vi "Carica lista canali.vi"(9 "BANCO":i32, 10 "LINEA":i32, 11 "Array":refnum<vi>[](array[refnum])) -> (0 "error out":errorcluster)   [LabVIEW 2019]
uses:
  <vilib>/Utility/file.llb/Read Delimited Spreadsheet (string).vi
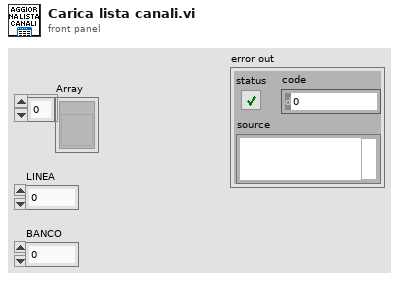
[diagram p1: front panel]
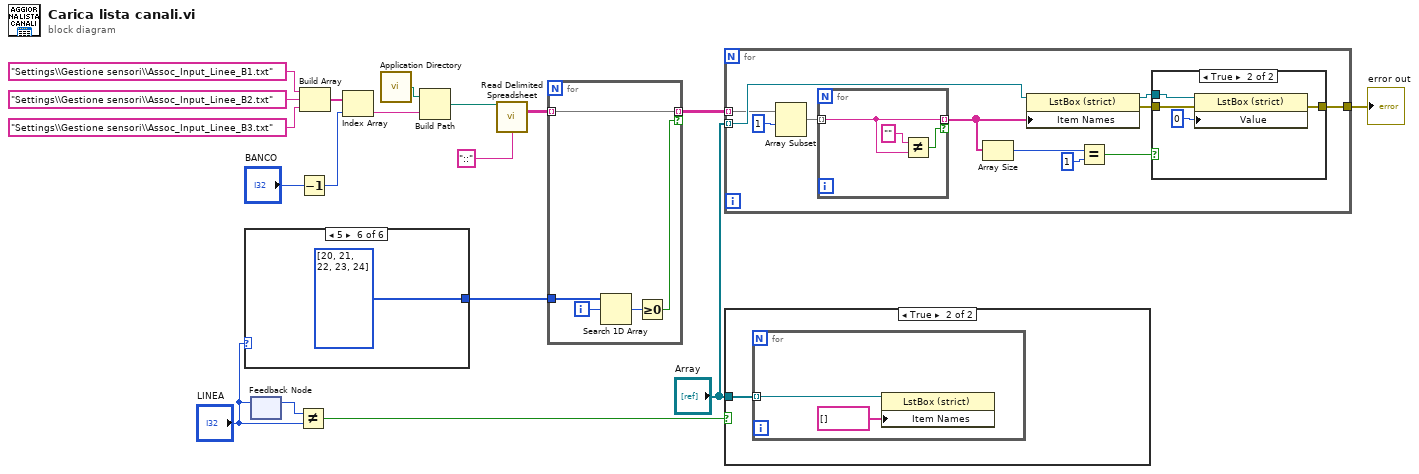
[diagram p0: block diagram]
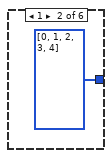
[diagram p4: hidden frame]
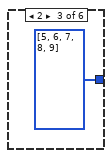
[diagram p5: hidden frame]
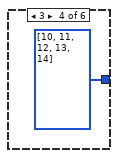
[diagram p6: hidden frame]
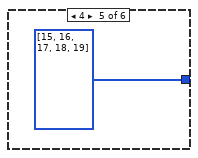
[diagram p7: hidden frame]
diagram:
  n1 = case shown="5" "LINEA" {
    tunnel: [_ i32[] [0, 1, 2, 3, 4] i32[] [5, 6, 7, 8, 9] i32[] [10, 11, 12, 13, 14] i32[] [15, 16, 17, 18, 19] i32[] [20, 21, 22, 23, 24]] -> w2
    frame 0, Default {
    }
    frame 1 {
    }
    frame 2 {
    }
    frame 3 {
    }
    frame 4 {
    }
    frame 5 {
    }
  }
  n2 = feedback-in #1("LINEA") -> ()
  n3 = feedback #1() -> (w7:i32)  [unwired: 1 in]
  n4 = Not Equal?(x=w7, y="LINEA") -> (x != y?=w5:bool)
  n5 = Decrement(x="BANCO") -> (x-1=w17:i32)
  n6 = Build Array("Settings\\Gestione sensori\\Assoc_Input_Linee_B1.txt" ("name or relative path"), "Settings\\Gestione sensori\\Assoc_Input_Linee_B2.txt" ("name or relative path"), "Settings\\Gestione sensori\\Assoc_Input_Linee_B3.txt" ("name or relative path")) -> (w10:string[])
  n7 = Index Array(array=w10, index=w17) -> (element=w14:string)
  n8 = call <vilib>:"Application Directory.vi"() -> ("Application Directory"=w13:path)
  n9 = Build Path(base path=w13, name or relative path=w14) -> (appended path=w15:path)
  n10 = call-poly <vilib>:"Read Delimited Spreadsheet.vi"("file path (dialog if empty)"=w15, "delimiter (\\t)"="::" ("delimiter (\\t)")) -> ("all rows"=w3:string[][])  [unwired: 8 in, 5 out]
  n11 = for {
    tunnel: w3 -> [w28] mode=indexing
    tunnel: [w28] -> w1 mode=indexing if=w24
    tunnel: w2 -> [w27]
    i -> [w26]
    n12 = Search 1D Array(1D array=w27, element=w26) -> (index of element=w25:i32)  [unwired: 1 in]
    n13 = Greater Or Equal To 0?(x=w25) -> (x >= 0?=w24:bool)
  }
  n14 = for {
    tunnel: "Array" -> [w39] mode=indexing
    tunnel: w1 -> [w38] mode=indexing
    tunnel: [w36] -> w4
    n15 = Array Subset(array=w38, index=1) -> (w35:string[])  [unwired: 1 in]
    n16 = for {
      tunnel: w35 -> [w46] mode=indexing
      tunnel: [w46] -> w34 mode=indexing if=w45
      n17 = Not Equal?(x="", y=w46) -> (x != y?=w45:bool)
    }
    n18 = Array Size(array=w34) -> (size(s)=w33:i32)
    n19 = property class="LstBox (strict)"(reference=w39, "Item Names"=w34) -> (reference out=w31:refnum<vi>, error out=w30:errorcluster)  [unwired: 1 in]
    n20 = Equal?(x=w33, y=1) -> (x = y?=w29:bool)
    n21 = case shown="True" w29 {
      tunnel: w31 -> [_ w44]
      tunnel: w30 -> [w40 w43]
      tunnel: [w40 w42] -> w36
      frame False {
      }
      frame True {
        n22 = property class="LstBox (strict)"(reference=w44, error in=w43, "Value"=0) -> (error out=w42:errorcluster)  [unwired: 1 out]
      }
    }
  }
  "error out" <- w4
  n23 = case shown="True" w5 {
    tunnel: "Array" -> [_ w48]
    frame False {
    }
    frame True {
      n24 = for {
        tunnel: w48 -> [w50] mode=indexing
        n25 = property class="LstBox (strict)"(reference=w50, "Item Names"=string[] []) -> ()  [unwired: 1 in, 2 out]
      }
    }
  }
